vi "CoordSystem_New.vi"(9 "PositiveZ":T1={"Axis"=[0.0, 0.0, 0.0]}, 10 "PositveY":T1={"Axis"=[0.0, 0.0, 0.0]}, 11 "PositiveX":T1={"Axis"=[0.0, 0.0, 0.0]}) -> (0 "Error":bool, 3 "out Coordinate System":T2={"Rotation"={"Q_quaternion"={"R"=1.0, "V"=[0.0, 0.0, 0.0]}}})   [LabVIEW 2019, in "Trajectory_Library.lvlib"]
doc: "Construct a Coordinte System data cluster which converts Pose3d objects between different standard coordinate frames. Contains a coordinate system with the given cardinal directions for each axis.\n\nInputs::\n -- PositiveX -- The cardinal direction of the positive x-axis.\n -- PositiveY -- The cardinal direction of the positive y-axis.\n -- PositiveZ -- The cardinal direction of the positive z-axis.\n\nReturns:\n -- out Coordinate System -- Data cluster containing the Coordinate System\n -- Error -- TRUE indicates an error occured."
uses:
  Trajectory_Library.lvlib
  TypeDef/COORDINATE_SYSTEM.ctl
  TypeDef/ROTATION3D.ctl
  TypeDef/QUATERNION.ctl
  TypeDef/COORDINATE_AXIS.ctl
  <vilib>/Analysis/baseanly.llb/Real A x B.vi
  MatrixHelper_CoerceSize.vi
  Quaternion_Normalize.vi
  Quaternion_New_Default.vi
  <vilib>/Analysis/7linalg.llb/Create Special Matrix.vi
  <vilib>/Analysis/7linalg.llb/Create Special Real Matrix.vi
  <vilib>/Analysis/Matrix/Numeric/Conversions/Array To Matrix - RA.vi
  <vilib>/Analysis/Matrix/NI_Matrix.lvlib
  <vilib>/Analysis/NI_AALBase.lvlib
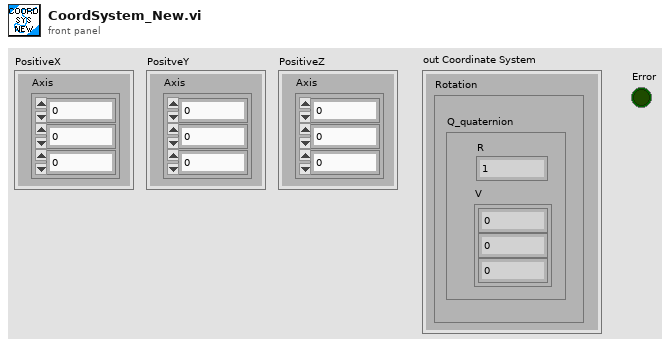
[diagram p1: front panel]
types:
  T1 = typedef "Trajectory_Library.lvlib/COORDINATE_AXIS.ctl" = cluster{"Axis":dbl[]}
  T2 = typedef "Trajectory_Library.lvlib/COORDINATE_SYSTEM.ctl" = cluster{"Rotation":T3}
  T3 = typedef "Trajectory_Library.lvlib/ROTATION3D.ctl" = cluster{"Q_quaternion":T4}
  T4 = typedef "Trajectory_Library.lvlib/QUATERNION.ctl" = cluster{"R":dbl, "V":dbl[]}
  T5 = typedef "NI_Matrix.lvlib/RealMatrix.ctl" = dbl[][]
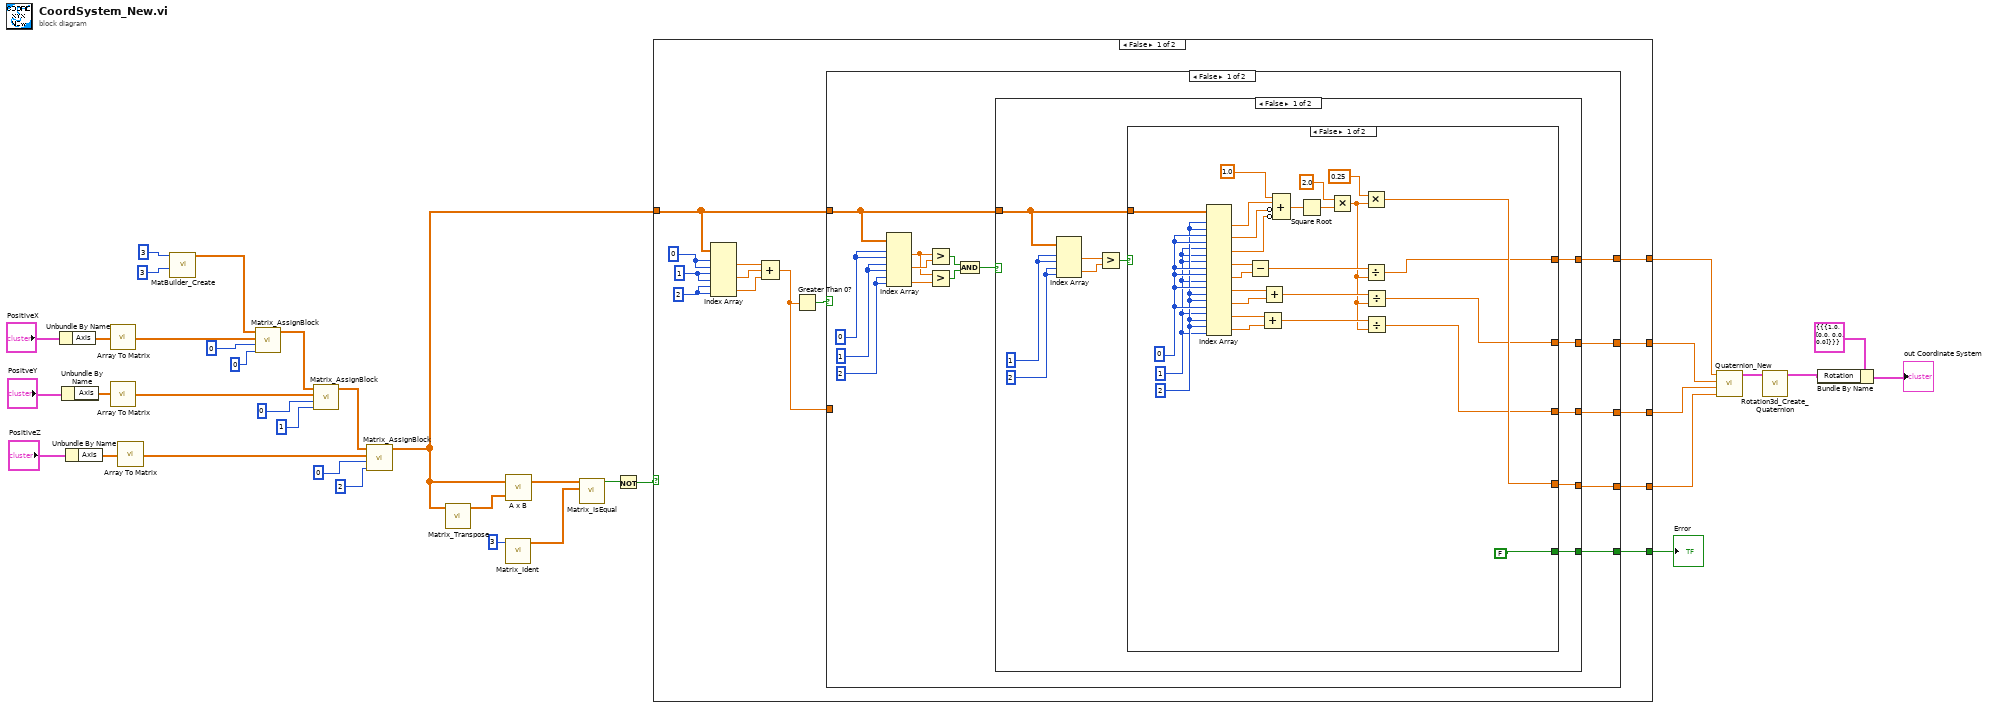
[diagram p0: block diagram]
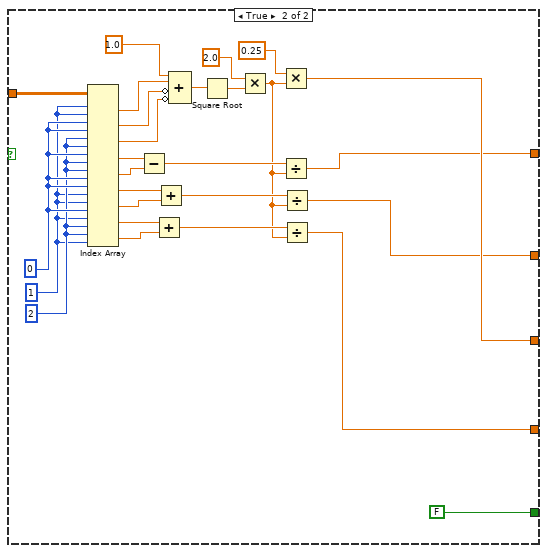
[diagram p2: hidden frame]
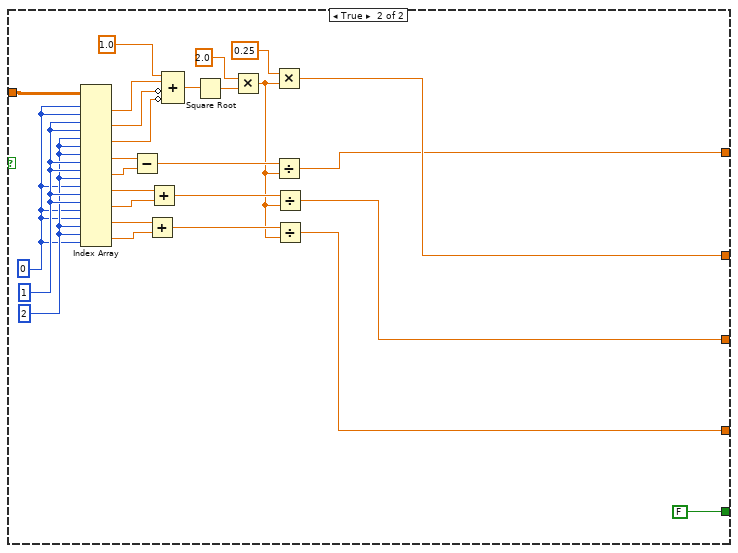
[diagram p3: hidden frame]
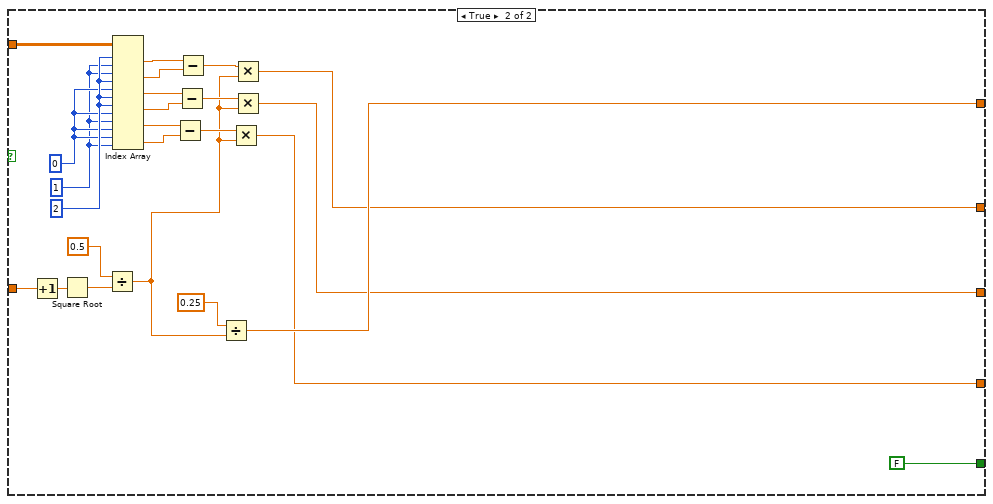
[diagram p4: hidden frame]
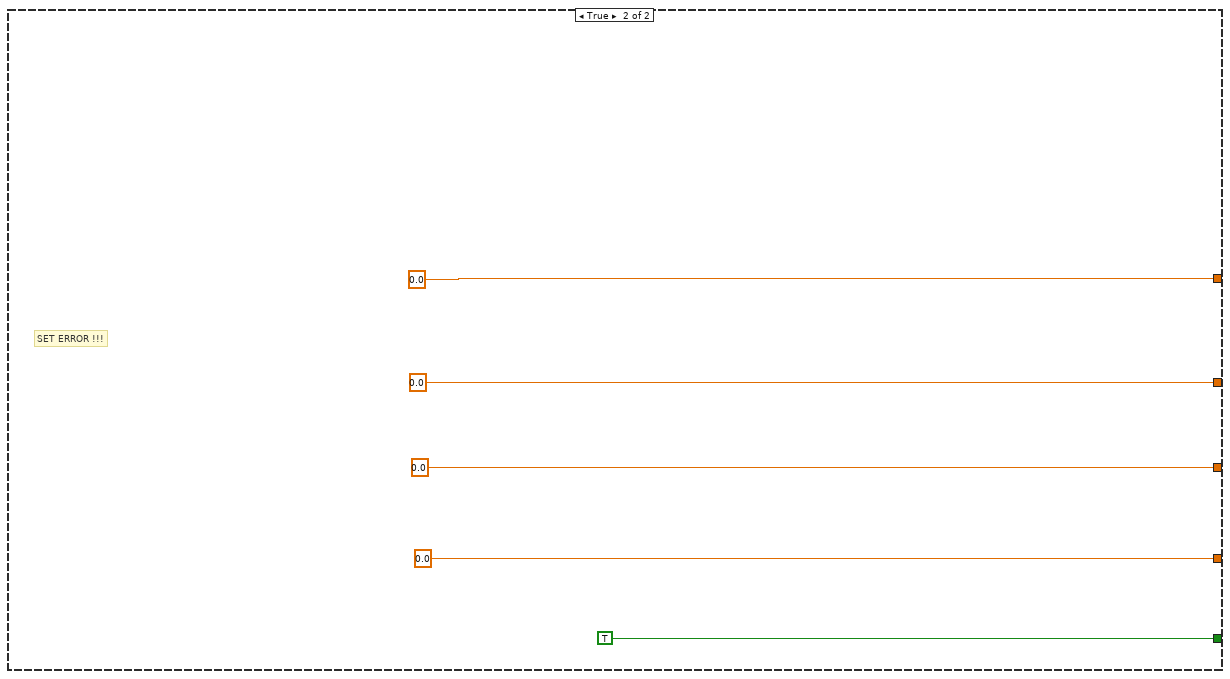
[diagram p5: hidden frame]
diagram:
  n1 = Unbundle By Name("PositiveX") -> ("Axis"=w26:dbl[])
  n2 = Unbundle By Name("PositveY") -> ("Axis"=w25:dbl[])
  n3 = Unbundle By Name("PositiveZ") -> ("Axis"=w24:dbl[])
  n4 = call-poly <vilib>:"Array To Matrix.vi"("Real 1D Array"=w26) -> ("Real Matrix (Column Vector)"=w23:T5)
  n5 = call-poly <vilib>:"Array To Matrix.vi"("Real 1D Array"=w25) -> ("Real Matrix (Column Vector)"=w22:T5)
  n6 = call-poly <vilib>:"Array To Matrix.vi"("Real 1D Array"=w24) -> ("Real Matrix (Column Vector)"=w21:T5)
  n7 = call "MatBuilder_Create.vi"("Columns"=3, "Rows"=3) -> ("output matrix"=w32:T5)  [unwired: 9 in]
  n8 = call "Matrix_AssignBlock.vi"("StartColumn"=0, "StartRow"=0, "Other Matrix"=w23, "input matrix"=w32) -> ("output matrix"=w31:T5)  [unwired: 7 in]
  n9 = call "Matrix_AssignBlock.vi"("StartColumn"=1, "StartRow"=0, "Other Matrix"=w22, "input matrix"=w31) -> ("output matrix"=w30:T5)  [unwired: 7 in]
  n10 = call "Matrix_AssignBlock.vi"("StartColumn"=2, "StartRow"=0, "Other Matrix"=w21, "input matrix"=w30) -> ("output matrix"=w2:T5)  [unwired: 7 in]
  n11 = call "Matrix_Transpose.vi"("input matrix"=w2) -> ("output matrix"=w13:T5)  [unwired: 10 in]
  n12 = call "Matrix_Ident.vi"("Size"=3) -> ("output matrix"=w14:T5)  [unwired: 9 in, 1 out]
  n13 = call-poly <vilib>:"A x B.vi"("B"=w13, "A"=w2) -> ("A x B"=w12:T5)  [unwired: 1 out]
  n14 = call "Matrix_IsEqual.vi"("other"=w14, "input matrix"=w12) -> ("Equal"=w10:bool)  [unwired: 9 in]
  n15 = Not(x=w10) -> (.not. x?=w9:bool)
  n16 = case shown="False" w9 {
    tunnel: [w41 0.0] -> w6
    tunnel: [w40 0.0] -> w5
    tunnel: [w39 0.0] -> w4
    tunnel: [w38 0.0] -> w3
    tunnel: w2 -> [w42 _]
    tunnel: [w37 TRUE] -> w1
    frame False {
      w48 = 2 ("index (row)")
      w49 = 1 ("index (row)")
      w50 = 0 ("index (row)")
      n17 = Index Array(array=w42, index (row) #1=w50, index (col) #1=w50, index (row) #2=w49, index (col) #2=w49, index (row) #3=w48, index (col) #3=w48) -> (element #1=w47:dbl, element #2=w46:dbl, element #3=w45:dbl)
      n18 = Compound Arithmetic op=ADD(w47, w46, w45) -> (w43:dbl)
      n19 = Greater Than 0?(x=w43) -> (x > 0?=w44:bool)
      n20 = case shown="False" w44 {
        tunnel: w43 -> [_ w181]
        tunnel: w42 -> [w65 w177]
        tunnel: [w54 w175] -> w41
        tunnel: [w55 w161] -> w40
        tunnel: [w53 w160] -> w39
        tunnel: [w52 w159] -> w38
        tunnel: [w51 FALSE] -> w37
        frame False {
          w61 = 2 ("index (row)")
          w63 = 1 ("index (row)")
          w64 = 0 ("index (row)")
          n21 = Index Array(array=w65, index (row) #1=w64, index (col) #1=w64, index (row) #2=w63, index (col) #2=w63, index (row) #3=w61, index (col) #3=w61) -> (element #1=w60:dbl, element #2=w62:dbl, element #3=w59:dbl)
          n22 = Greater?(x=w60, y=w62) -> (0:w57:bool)
          n23 = Greater?(x=w60, y=w59) -> (0:w58:bool)
          n24 = And(x=w57, y=w58) -> (x .and. y?=w56:bool)
          n25 = case shown="False" w56 {
            tunnel: w65 -> [w71 w157]
            tunnel: [w68 w148] -> w55
            tunnel: [w69 w144] -> w54
            tunnel: [w70 w133] -> w53
            tunnel: [w67 w132] -> w52
            tunnel: [w66 FALSE] -> w51
            frame False {
              w73 = 2 ("index (row)")
              w74 = 1 ("index (row)")
              n26 = Index Array(array=w71, index (row) #1=w74, index (col) #1=w74, index (row) #2=w73, index (col) #2=w73) -> (element #1=w75:dbl, element #2=w76:dbl)
              n27 = Greater?(x=w75, y=w76) -> (0:w72:bool)
              n28 = case shown="False" w72 {
                tunnel: w71 -> [w85 w112]
                tunnel: [w78 w111] -> w70
                tunnel: [w80 w107] -> w69
                tunnel: [w79 w106] -> w68
                tunnel: [w84 w105] -> w67
                tunnel: [FALSE FALSE] -> w66
                frame False {
                  w82 = 2 ("index (row)")
                  w81 = 1 ("index (row)")
                  w83 = 0 ("index (row)")
                  n29 = Index Array(array=w85, index (row) #1=w82, index (col) #1=w82, index (row) #2=w83, index (col) #2=w83, index (row) #3=w81, index (col) #3=w81, index (row) #4=w81, index (col) #4=w83, index (row) #5=w83, index (col) #5=w81, index (row) #6=w83, index (col) #6=w82, index (row) #7=w82, index (col) #7=w83, index (row) #8=w81, index (col) #8=w82, index (row) #9=w82, index (col) #9=w81) -> (element #1=w102:dbl, element #2=w101:dbl, element #3=w100:dbl, element #4=w95:dbl, element #5=w94:dbl, element #6=w92:dbl, element #7=w91:dbl, element #8=w90:dbl, element #9=w89:dbl)
                  n30 = Subtract ("Subtract.vi")(x=w95, y=w94) -> (x-y=w93:dbl)
                  n31 = Add ("Add.vi")(x=w90, y=w89) -> (x+y=w88:dbl)
                  n32 = Add ("Add.vi")(x=w92, y=w91) -> (x+y=w87:dbl)
                  n33 = Compound Arithmetic op=ADD(1.0, w102, invert w101, invert w100) -> (w99:dbl)
                  n34 = Square Root(x=w99) -> (sqrt(x)=w98:dbl)
                  n35 = Multiply(x=2.0, y=w98) -> (x*y=w86:dbl)
                  n36 = Multiply(x=0.25, y=w86) -> (x*y=w84:dbl)
                  n37 = Divide(x=w93, y=w86) -> (x/y=w80:dbl)
                  n38 = Divide(x=w87, y=w86) -> (x/y=w79:dbl)
                  n39 = Divide(x=w88, y=w86) -> (x/y=w78:dbl)
                }
                frame True {
                  w109 = 2 ("index (row)")
                  w108 = 1 ("index (row)")
                  w110 = 0 ("index (row)")
                  n40 = Index Array(array=w112, index (row) #1=w108, index (col) #1=w108, index (row) #2=w110, index (col) #2=w110, index (row) #3=w109, index (col) #3=w109, index (row) #4=w110, index (col) #4=w109, index (row) #5=w109, index (col) #5=w110, index (row) #6=w110, index (col) #6=w108, index (row) #7=w108, index (col) #7=w110, index (row) #8=w108, index (col) #8=w109, index (row) #9=w109, index (col) #9=w108) -> (element #1=w129:dbl, element #2=w128:dbl, element #3=w127:dbl, element #4=w122:dbl, element #5=w121:dbl, element #6=w119:dbl, element #7=w118:dbl, element #8=w117:dbl, element #9=w116:dbl)
                  n41 = Subtract ("Subtract.vi")(x=w122, y=w121) -> (x-y=w120:dbl)
                  n42 = Add ("Add.vi")(x=w117, y=w116) -> (x+y=w115:dbl)
                  n43 = Add ("Add.vi")(x=w119, y=w118) -> (x+y=w114:dbl)
                  n44 = Compound Arithmetic op=ADD(1.0, w129, invert w128, invert w127) -> (w126:dbl)
                  n45 = Square Root(x=w126) -> (sqrt(x)=w125:dbl)
                  n46 = Multiply(x=2.0, y=w125) -> (x*y=w113:dbl)
                  n47 = Multiply(x=0.25, y=w113) -> (x*y=w111:dbl)
                  n48 = Divide(x=w120, y=w113) -> (x/y=w107:dbl)
                  n49 = Divide(x=w114, y=w113) -> (x/y=w106:dbl)
                  n50 = Divide(x=w115, y=w113) -> (x/y=w105:dbl)
                }
              }
            }
            frame True {
              w142 = 2 ("index (row)")
              w143 = 1 ("index (row)")
              w141 = 0 ("index (row)")
              n51 = Index Array(array=w157, index (row) #1=w141, index (col) #1=w141, index (row) #2=w143, index (col) #2=w143, index (row) #3=w142, index (col) #3=w142, index (row) #4=w142, index (col) #4=w143, index (row) #5=w143, index (col) #5=w142, index (row) #6=w141, index (col) #6=w143, index (row) #7=w143, index (col) #7=w141, index (row) #8=w141, index (col) #8=w142, index (row) #9=w142, index (col) #9=w141) -> (element #1=w155:dbl, element #2=w154:dbl, element #3=w153:dbl, element #4=w147:dbl, element #5=w146:dbl, element #6=w140:dbl, element #7=w139:dbl, element #8=w138:dbl, element #9=w137:dbl)
              n52 = Subtract(x=w147, y=w146) -> (x-y=w145:dbl)
              n53 = Add(x=w138, y=w137) -> (x+y=w136:dbl)
              n54 = Add(x=w140, y=w139) -> (x+y=w135:dbl)
              n55 = Compound Arithmetic op=ADD(1.0, w155, invert w154, invert w153) -> (w152:dbl)
              n56 = Square Root(x=w152) -> (sqrt(x)=w151:dbl)
              n57 = Multiply(x=2.0, y=w151) -> (x*y=w134:dbl)
              n58 = Multiply(x=0.25, y=w134) -> (x*y=w148:dbl)
              n59 = Divide(x=w145, y=w134) -> (x/y=w144:dbl)
              n60 = Divide(x=w135, y=w134) -> (x/y=w133:dbl)
              n61 = Divide(x=w136, y=w134) -> (x/y=w132:dbl)
            }
          }
        }
        frame True {
          w172 = 2 ("index (row)")
          w170 = 1 ("index (row)")
          w171 = 0 ("index (row)")
          n62 = Increment(x=w181) -> (x+1=w180:dbl)
          n63 = Square Root(x=w180) -> (sqrt(x)=w179:dbl)
          n64 = Divide(x=0.5, y=w179) -> (x/y=w162:dbl)
          n65 = Index Array(array=w177, index (row) #1=w172, index (col) #1=w170, index (row) #2=w170, index (col) #2=w172, index (row) #3=w171, index (col) #3=w172, index (row) #4=w172, index (col) #4=w171, index (row) #5=w170, index (col) #5=w171, index (row) #6=w171, index (col) #6=w170) -> (element #1=w174:dbl, element #2=w173:dbl, element #3=w169:dbl, element #4=w168:dbl, element #5=w167:dbl, element #6=w166:dbl)
          n66 = Subtract(x=w167, y=w166) -> (x-y=w163:dbl)
          n67 = Subtract(x=w169, y=w168) -> (x-y=w164:dbl)
          n68 = Subtract(x=w174, y=w173) -> (x-y=w165:dbl)
          n69 = Divide(x=0.25, y=w162) -> (x/y=w175:dbl)
          n70 = Multiply(x=w163, y=w162) -> (x*y=w159:dbl)
          n71 = Multiply(x=w165, y=w162) -> (x*y=w161:dbl)
          n72 = Multiply(x=w164, y=w162) -> (x*y=w160:dbl)
        }
      }
    }
    frame True {
      # "SET ERROR !!!"
    }
  }
  "Error" <- w1
  n73 = call "Quaternion_New.vi"("Z"=w3, "Y"=w4, "X"=w5, "W"=w6) -> ("out Quaternion"=w8:T4)  [unwired: 7 in]
  n74 = call "Rotation3d_Create_Quaternion.vi"("Quaternion"=w8) -> ("Rotation3d"=w7:T3)  [unwired: 10 in]
  n75 = Bundle By Name(cluster=T2 {"Rotation"={"Q_quaternion"={"R"=1.0, "V"=[0.0, 0.0, 0.0]}}} ("sumPOSE"), "Rotation"=w7) -> (→"out Coordinate System":T2)
